vi "Remove_FF_lone_spikes.vi"(3 "ADC Frequency Hz":dbl=1000.0 format="%.2f", 4 "Bkgnd variance":dbl format="%.6f", 5 "Analysis Info cluster":T1={"Colour"=0, "Inst type"=enum."Pitot-static tube", "Inst name"="Manometer voltage", "Symbol"="U", "Code name"="", "Extra Info"="U", "Inst Array"=enum."PWA", "Index"=0, "Voltage Index"=0, "Extra Titles"=[], "Extra Values"=[]}, 6 "Time Trace":dbl[](graph)) -> (0 "No Removed":i32, 1 "Analysis Info cluster out":T1={"Colour"=0, "Inst type"=enum."Pitot-static tube", "Inst name"="Manometer voltage", "Symbol"="U", "Code name"="", "Extra Info"="U", "Inst Array"=enum."PWA", "Index"=0, "Voltage Index"=0, "Extra Titles"=[], "Extra Values"=[]}, 2 "Filtered Time Trace":dbl[](graph))   [LabVIEW 2010]
uses:
  Controls/Analysis_info_cluster.ctl
  Controls/Inst_type.ctl
  Controls/Instrument_Array.ctl
  Globals/Meas_global.vi
  <vilib>/Analysis/NI_AALBase.lvlib
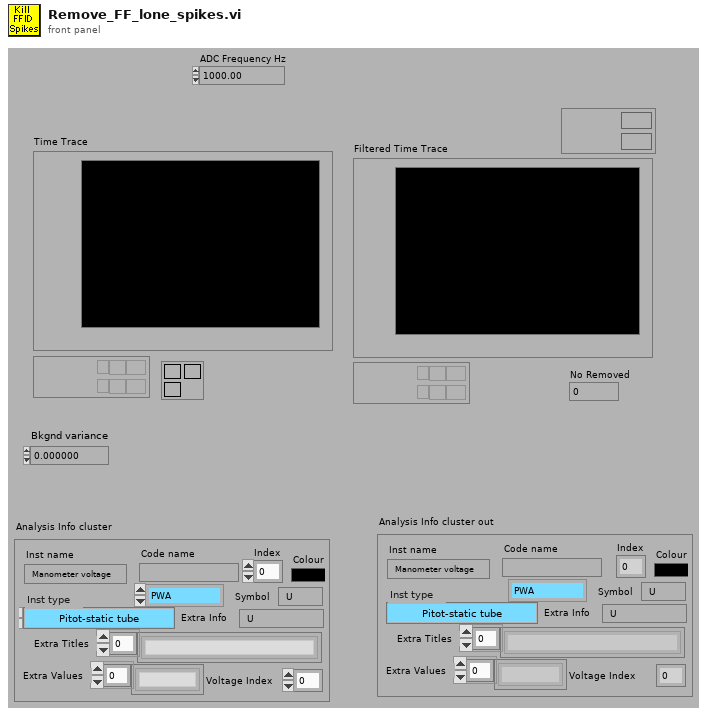
[diagram p1: front panel]
types:
  T1 = typedef "Analysis_info_cluster.ctl" = cluster{"Colour":u32, "Inst type":T2, "Inst name":string, "Symbol":string, "Code name":string, "Extra Info":string, "Inst Array":T3, "Index":i32, "Voltage Index":i32, "Extra Titles":string[], "Extra Values":string[]}
  T2 = typedef "Inst_type.ctl" = enum16{"Propeller anemometer", "Raw voltage", "Pressure Transducer", "Pitot-static tube", "Preston tube", "Hot wire", "Cross wire 1", "Cross wire 2", "Generic Linear", "Generic Polynomial", "Generic BackPoly", "Fast FID", "Thermocouple", "Cold wire", "Pulsed Wire", "LDA Vel", "LDA Tran time", "LDA Arr time"}
  T3 = typedef "Instrument_Array.ctl" = enum16{"PWA", "LDA", "Analogue"}
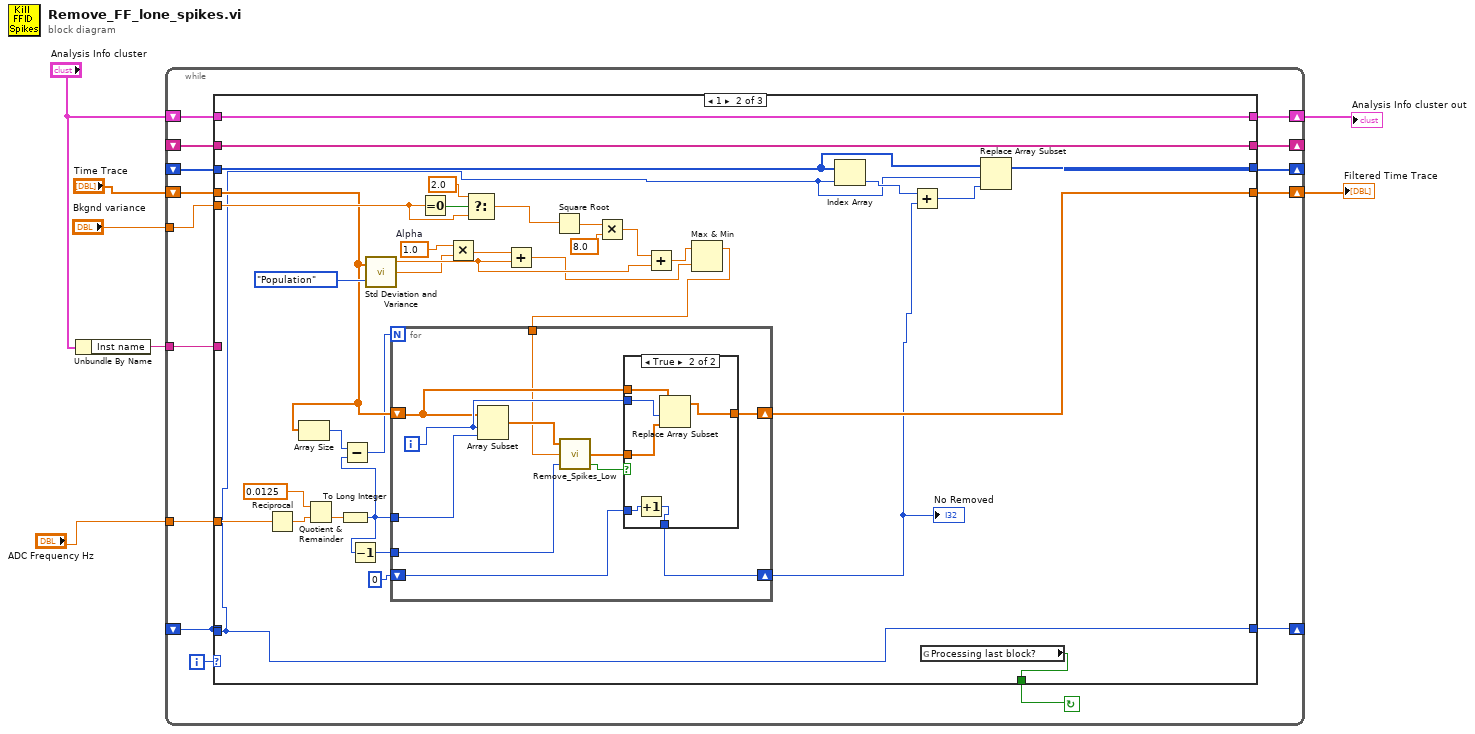
[diagram p0: block diagram]
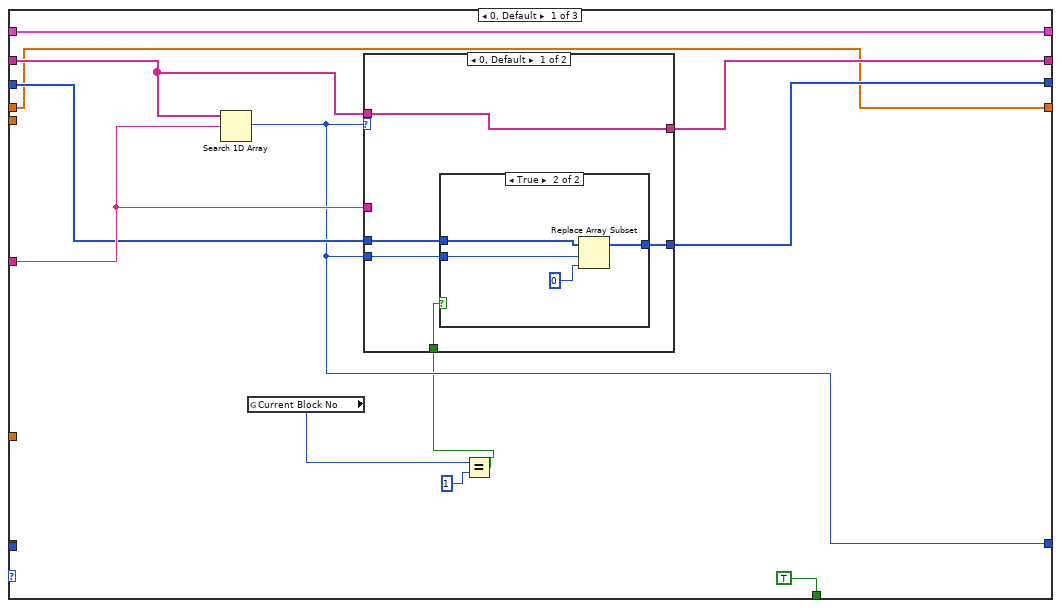
[diagram p2: hidden frame]
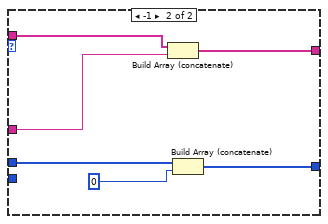
[diagram p4: hidden frame]
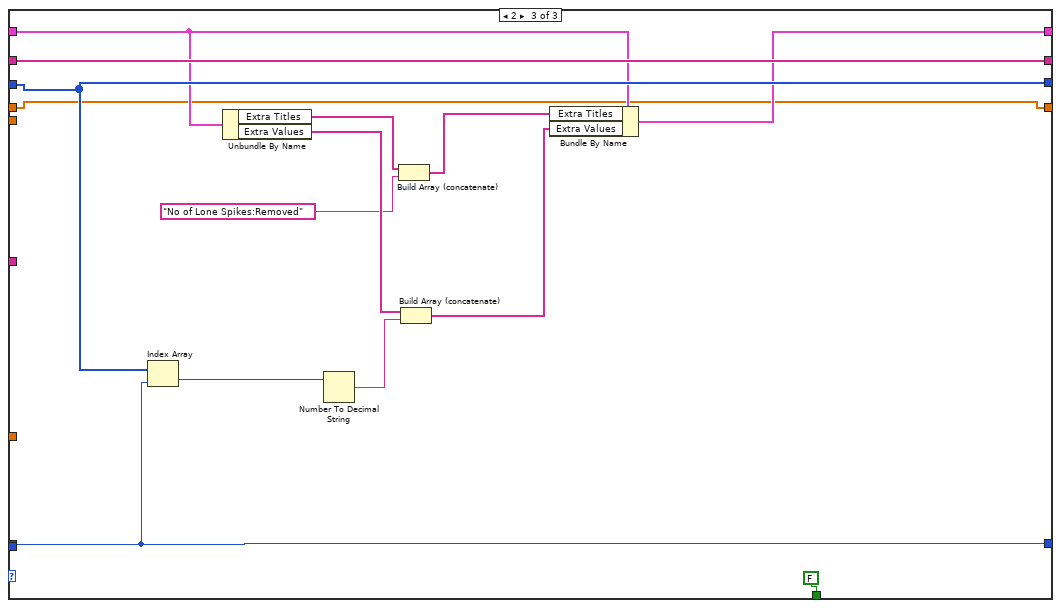
[diagram p6: hidden frame]
diagram:
  n1 = Unbundle By Name("Analysis Info cluster") -> ("Inst name"=w7:string)
  n2 = while {
    shift-left: _ -> [w19]
    shift-right: [w21] -> _
    tunnel: w7 -> [w18]
    shift-right: [w16] -> _
    shift-left: _ -> [w17]
    shift-right: [w14] -> _
    shift-left: _ -> [w15]
    shift-right: [w12] -> w5
    shift-left: "Analysis Info cluster" -> [w13]
    tunnel: "Bkgnd variance" -> [w11]
    shift-right: [w9] -> w2
    shift-left: "Time Trace" -> [w10]
    tunnel: "ADC Frequency Hz" -> [w8]
    i -> [w22]
    stop <- w20 continue-if-true
    n3 = case shown="1" w22 {
      tunnel: [w26 w55 w116] -> w21
      tunnel: [TRUE w53 FALSE ("Processing last block?")] -> w20
      tunnel: w19 -> [_ _ w116]
      tunnel: w19 -> [_ w55 _]
      tunnel: w18 -> [w30 _ _]
      tunnel: w17 -> [w31 w73 w114]
      tunnel: [w29 w73 w114] -> w16
      tunnel: w15 -> [w28 w72 w113]
      tunnel: [w27 w70 w113] -> w14
      tunnel: w13 -> [w24 w69 w110]
      tunnel: [w24 w69 w112] -> w12
      tunnel: w11 -> [_ w67 _]
      tunnel: w10 -> [w23 w60 w105]
      tunnel: [w23 w54 w105] -> w9
      tunnel: w8 -> [_ w65 _]
      frame 0, Default {
        n4 = Search 1D Array(1D array=w31, element=w30) -> (index of element=w26:i32)  [unwired: 1 out]
        n5 = global read "Meas_global.vi" "Current Block No"() -> (w33:i32)
        n6 = Equal?(x=w33, y=1) -> (x = y?=w25:bool)
        n7 = case shown="0, Default" w26 {
          tunnel: w31 -> [w39 w50]
          tunnel: w30 -> [_ w49]
          tunnel: [w39 w48] -> w29
          tunnel: w28 -> [w38 w47]
          tunnel: [w37 w46] -> w27
          tunnel: w26 -> [w36 _]
          tunnel: w25 -> [w35 _]
          frame 0, Default {
            n8 = case shown="True" w35 {
              tunnel: w38 -> [w40 w44]
              tunnel: [w40 w43] -> w37
              tunnel: w36 -> [_ w42]
              frame False {
              }
              frame True {
                n9 = Replace Array Subset(array=w44, new element=0, index=w42) -> (w43:i32[])
              }
            }
          }
          frame -1 {
            n10 = Build Array (concatenate)(w50, w49) -> (w48:string[])
            n11 = Build Array (concatenate)(w47, 0) -> (w46:i32[])
          }
        }
      }
      frame 1 {
        w85 = 1.0  # Alpha
        n12 = Reciprocal(x=w65) -> (1/x=w63:dbl)
        n13 = Array Size(array=w60) -> (size(s)=w59:i32)
        n14 = Quotient & Remainder(x=0.0125, y=w63) -> (floor(x/y)=w62:dbl)  [unwired: 1 out]
        n15 = To Long Integer(number=w62) -> (32bit integer=w58:i32)
        n16 = Subtract(x=w59, y=w58) -> (x-y=w57:i32)
        n17 = Decrement(x=w58) -> (x-1=w61:i32)
        n18 = call <vilib>:"Std Deviation and Variance.vi"("X"=w60, "Weighting (Sample)"=enum16{"Sample", "Population"}."Population") -> ("mean"=w80:dbl, "standard deviation"=w68:dbl)  [unwired: 1 out]
        n19 = Equal To 0?(x=w67) -> (x = 0?=w79:bool)
        n20 = Multiply(x=w85, y=w68) -> (x*y=w84:dbl)
        n21 = Select(t=2.0, s=w79, f=w67) -> (s? t:f=w77:dbl)
        n22 = Add(x=w84, y=w80) -> (x+y=w74:dbl)
        n23 = Square Root(x=w77) -> (sqrt(x)=w83:dbl)
        n24 = Multiply(x=w83, y=8.0) -> (x*y=w81:dbl)
        n25 = Add(x=w81, y=w80) -> (x+y=w75:dbl)
        n26 = Max & Min(x=w75, y=w74) -> (max(x,y)=w56:dbl)  [unwired: 1 out]
        n27 = for {
          N: w57 -> [_]
          shift-right: [w89] -> w54
          shift-left: w60 -> [w90]
          tunnel: w58 -> [w96]
          tunnel: w61 -> [w95]
          tunnel: w56 -> [w88]
          shift-right: [w87] -> w52
          shift-left: 0 -> [w86]
          i -> [w92]
          n28 = Array Subset(array=w90, index=w92, length=w96) -> (w94:dbl[])
          n29 = call "Remove_Spikes_Low.vi"("index"=w95, "Background noise"=w88, "Time Trace"=w94) -> ("Spike"=w93:bool, "Filtered Time Trace"=w91:dbl[])  [unwired: 1 out]
          n30 = case shown="True" w93 {
            tunnel: w92 -> [_ w104]
            tunnel: w91 -> [_ w103]
            tunnel: w90 -> [w98 w102]
            tunnel: [w98 w101] -> w89
            tunnel: [w97 w99] -> w87
            tunnel: w86 -> [w97 w100]
            frame False {
            }
            frame True {
              n31 = Increment(x=w100) -> (x+1=w99:i32)
              n32 = Replace Array Subset(array=w102, new element=w103, index=w104) -> (w101:dbl[])
            }
          }
        }
        "No Removed" <- w52
        n33 = Index Array(array=w72, index=w55) -> (element=w71:i32)
        n34 = Add(x=w71, y=w52) -> (x+y=w66:i32)
        n35 = global read "Meas_global.vi" "Processing last block?"() -> (w53:bool)
        n36 = Replace Array Subset(array=w72, new element=w66, index=w55) -> (w70:i32[])
      }
      frame 2 {
        n37 = Index Array(array=w113, index=w116) -> (element=w115:i32)
        n38 = Unbundle By Name(w110) -> ("Extra Titles"=w109:string[], "Extra Values"=w108:string[])
        n39 = Number To Decimal String(number=w115) -> (decimal integer string=w117:string)  [unwired: 1 out]
        n40 = Build Array (concatenate)(w109, "No of Lone Spikes:Removed" ("format string")) -> (w111:string[])
        n41 = Build Array (concatenate)(w108, w117) -> (w107:string[])
        n42 = Bundle By Name(cluster=w110, "Extra Titles"=w111, "Extra Values"=w107) -> (w112:T1)
      }
    }
  }
  "Analysis Info cluster out" <- w5
  "Filtered Time Trace" <- w2
